vi "SubVI_Clamp #.vi"(8 "error in":errorcluster, 10 "Parameter_Edge":T3={"ROI Descriptor"={"Global Rectangle"=[], "Contours"=[]}, "Edge Options"={"Edge Options"={"Edge Polarity"=0, "Kernel Size"=3, "Width"=3, "Minimum Edge Strength"=10.0, "Interpolation Type"=enum."Bilinear Fixed", "Data Processing Method"=enum."Average"}, "Scan Direction"=0, "Step Size"=5, "SD"=0.0, "Auto"=FALSE}, "條件(Clamp)"={"間距"=5.0}} {"ROI Descriptor"."Contours"."Type" items=["No Selection", "Point", "Line", "Rectangle", "Oval", "Polygon", "Free", "Annulus", "Unused2", "Unused3", "Broken Line", "Free Hand Line", "Rotated Rectangle"]; "Edge Options"."Edge Options"."Edge Polarity" items=["All Edges", "Rising Edges", "Falling Edges"]; "Edge Options"."Edge Options"."Minimum Edge Strength" format="%.2f"; "Edge Options"."Edge Options"."Width" step=2; "Edge Options"."Edge Options"."Kernel Size" step=2; "Edge Options"."Scan Direction" items=["Left To Right", "Right To Left", "Top To Bottom", "Bottom To Top"]}, 11 "Image in":T2) -> (0 "error out":errorcluster, 1 "Distance":dbl, 2 "Perpendicular Line(Offset)":T1, 3 "Image Out":T2, 4 "Fit Line 2":T1, 6 "Fit Line":T1)   [LabVIEW 2013]
uses:
  <vilib>/vision/Image Controls.llb/IMAQ Image.ctl
  Control/Control_Clamp.ctl
  <vilib>/vision/Measure.llb/Edge Options.ctl
  <vilib>/vision/Measure.llb/Edge Polarity.ctl
  <vilib>/vision/NI_Vision_Development_Module.lvlib
  <vilib>/Analysis/NI_AALBase.lvlib
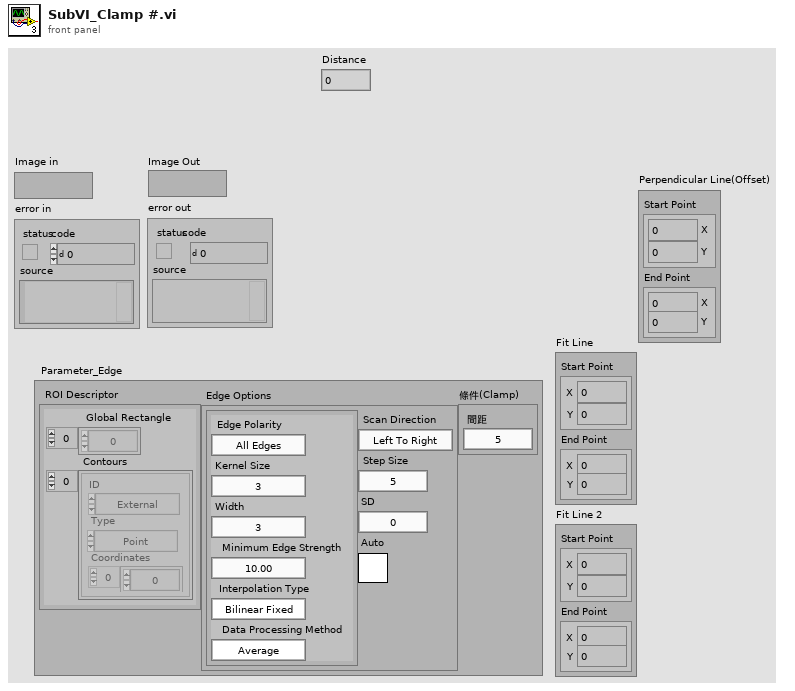
[diagram p1: front panel]
types:
  T1 = cluster{"Start Point":cluster{"X":sgl, "Y":sgl}, "End Point":cluster{"X":sgl, "Y":sgl}}
  T2 = typedef "IMAQ Image.ctl" = refnum<image>
  T3 = typedef "Control_Clamp.ctl" = cluster{"ROI Descriptor":cluster{"Global Rectangle":i32[], "Contours":cluster{"ID":enum32{"External", "Internal"}, "Type":u32, "Coordinates":i32[]}[]}, "Edge Options":cluster{"Edge Options":T4, "Scan Direction":u16, "Step Size":u32, "SD":dbl, "Auto":bool}, "條件(Clamp)":cluster{"間距":dbl}}
  T4 = typedef "Edge Options.ctl" = cluster{"Edge Polarity":T5, "Kernel Size":u32, "Width":u32, "Minimum Edge Strength":sgl, "Interpolation Type":enum32{"Zero Order", "Bilinear", "Quadratic", "Cubic", "Bilinear Fixed"}, "Data Processing Method":enum32{"Average", "Median"}}
  T5 = typedef "Edge Polarity.ctl" = u32
  T6 = cluster{"Global Rectangle":i32[], "Contours":cluster{"ID":enum32{"External", "Internal"}, "Type":u32, "Coordinates":i32[]}[]}
  T7 = cluster{"Edge Options":T4, "Scan Direction":u16, "Step Size":u32, "SD":dbl, "Auto":bool}
  T8 = cluster{"Point 1":cluster{"X":sgl, "Y":sgl}, "Point 2":cluster{"X":sgl, "Y":sgl}}
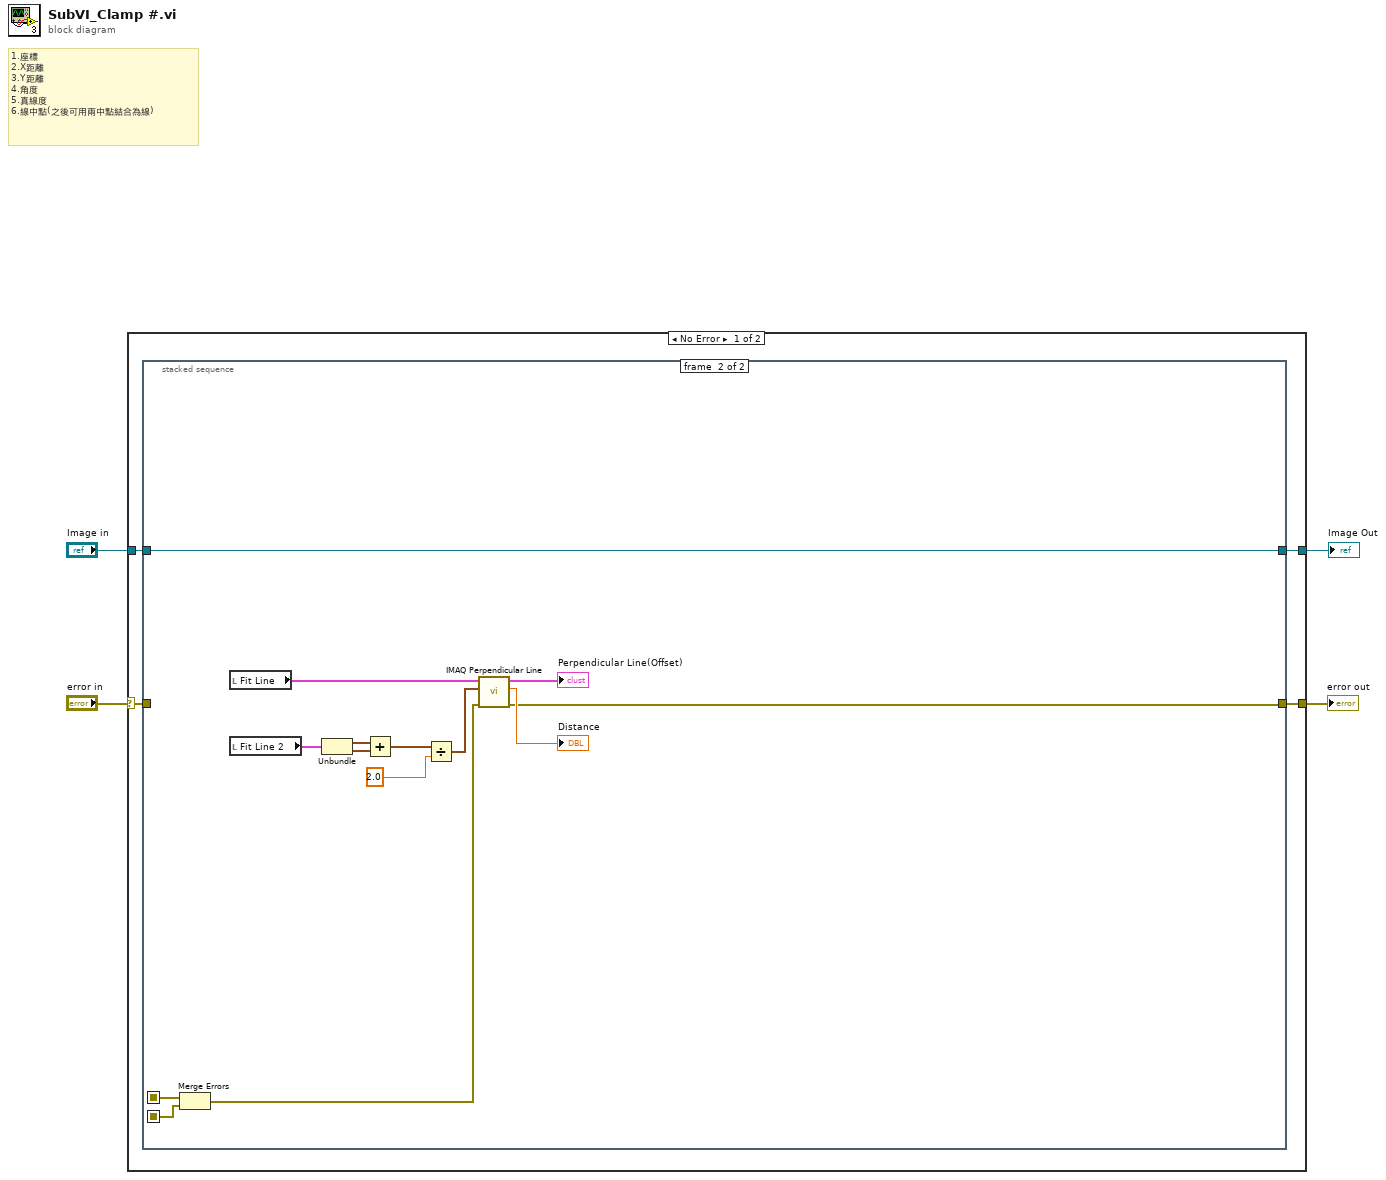
[diagram p0: block diagram]
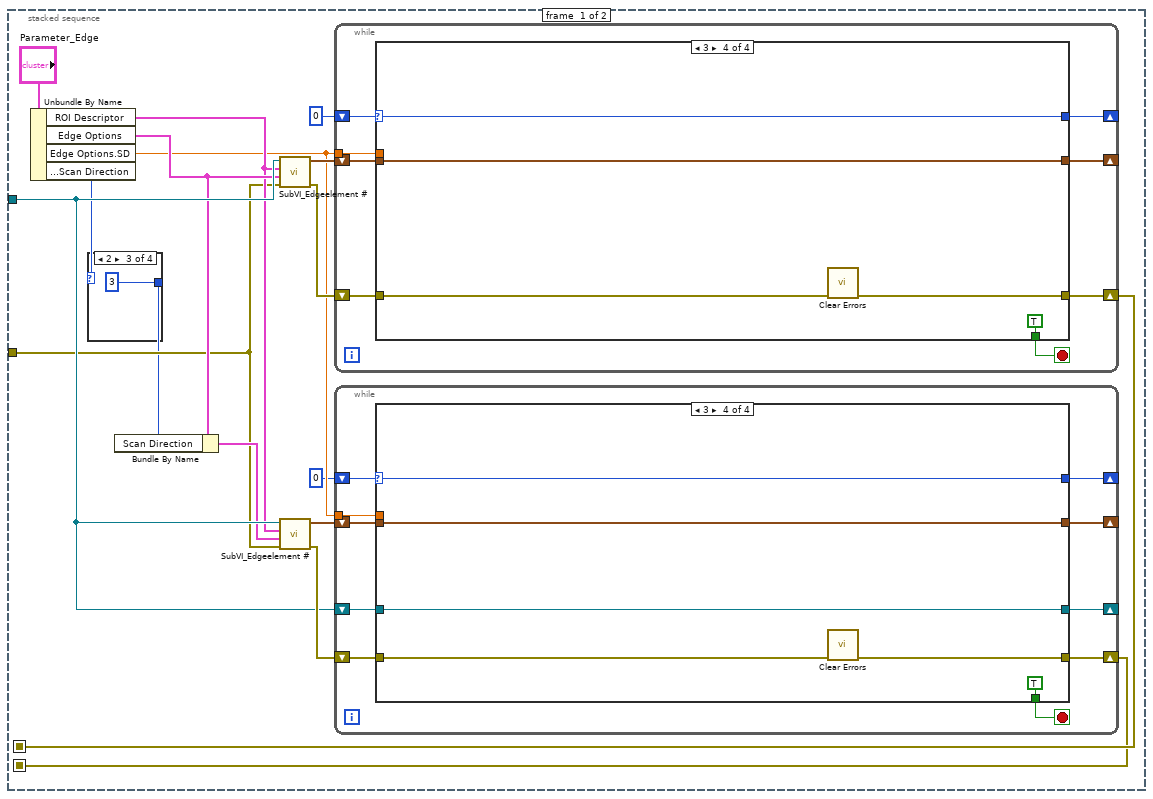
[diagram p2: hidden frame]
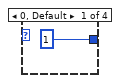
[diagram p3: hidden frame]
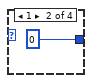
[diagram p4: hidden frame]
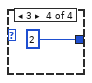
[diagram p5: hidden frame]
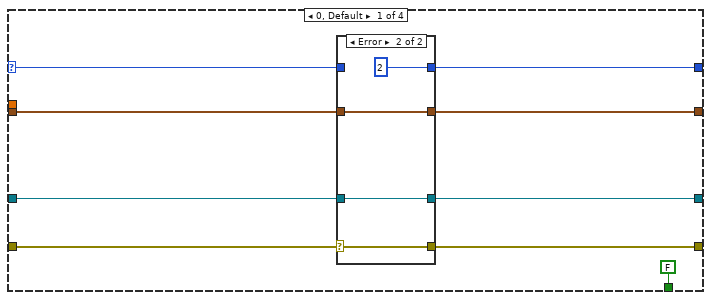
[diagram p6: hidden frame]
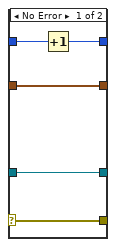
[diagram p7: hidden frame]
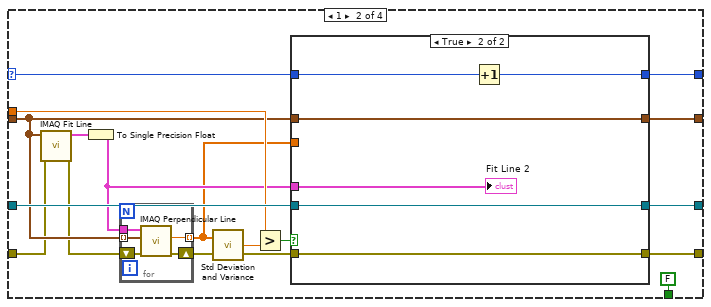
[diagram p8: hidden frame]
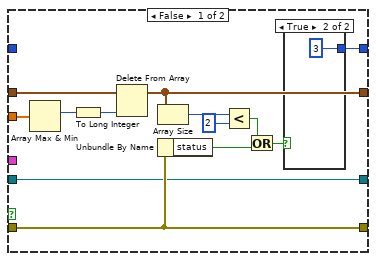
[diagram p9: hidden frame]
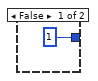
[diagram p10: hidden frame]
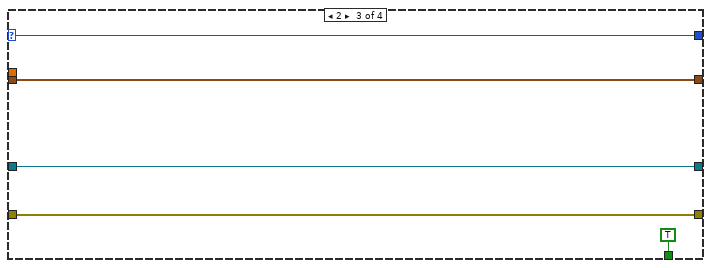
[diagram p11: hidden frame]
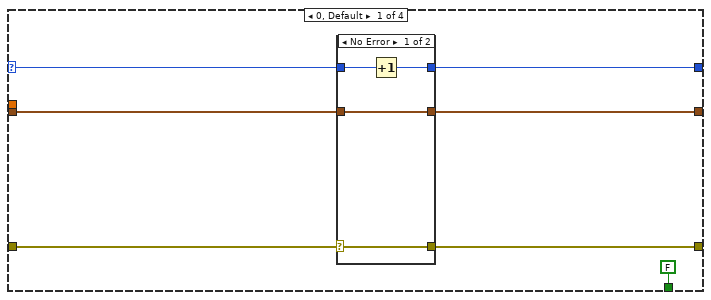
[diagram p12: hidden frame]
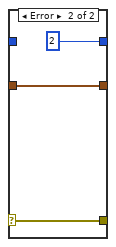
[diagram p13: hidden frame]
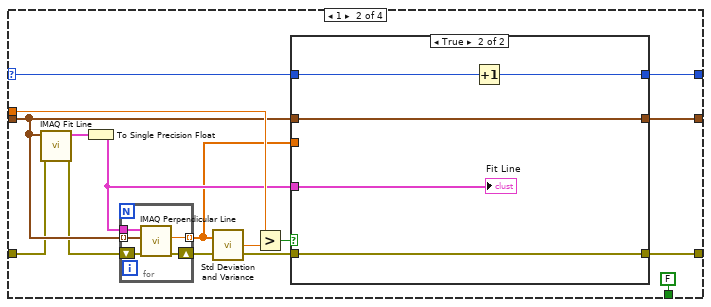
[diagram p14: hidden frame]
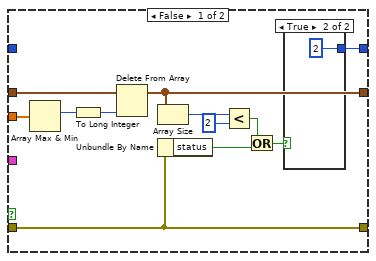
[diagram p15: hidden frame]
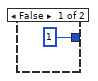
[diagram p16: hidden frame]
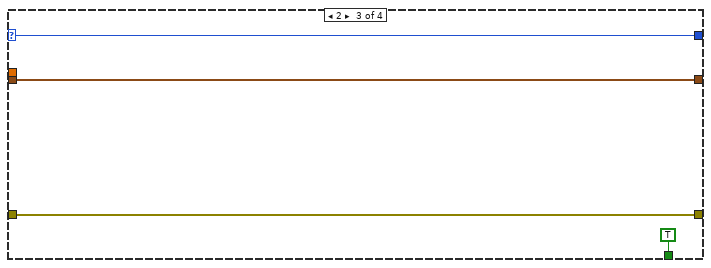
[diagram p17: hidden frame]
diagram:
  # "1.座標\n2.X距離\n3.Y距離\n4.角度\n5.真線度\n6.線中點(之後可用兩中點結合為線)"
  n1 = case shown="No Error" "error in" {
    selector: "error in" -> [w5 w197]
    tunnel: "Image in" -> [w6 w196]
    tunnel: [w8 w197] -> w2
    tunnel: [w7 w196] -> w1
    frame No Error {
      n2 = stacked-sequence {
        seq-local: [w10 _] -> [_ w184]
        seq-local: [w9 _] -> [_ w183]
        tunnel: [_ w185] -> w8
        tunnel: [_ w195] -> w7
        tunnel: w6 -> [w20 w195]
        tunnel: w5 -> [w16 _]
        frame #0 {
          n3 = Unbundle By Name("Parameter_Edge") -> ("ROI Descriptor"=w17:T6, "Edge Options"=w19:T7, "Edge Options.SD"=w13:dbl, "Edge Options.Scan Direction"=w15:u16)
          n4 = case shown="2" w15 {
            tunnel: [u16 1 u16 0 u16 3 u16 2] -> w14
            frame 0, Default {
            }
            frame 1 {
            }
            frame 2 {
            }
            frame 3 {
            }
          }
          n5 = Bundle By Name(cluster=w19, "Scan Direction"=w14) -> (w18:T7)
          n6 = call "SubVI_Edgeelement #.vi"("Error In"=w16, "Parameter_Edge"=w19, "ROI Descriptor"=w17, "Image In"=w20) -> ("Error Out"=w24:errorcluster, "Location"=w22:cluster{"X":sgl, "Y":sgl}[])  [unwired: 4 in, 2 out]
          n7 = call "SubVI_Edgeelement #.vi"("Error In"=w16, "Parameter_Edge"=w18, "ROI Descriptor"=w17, "Image In"=w20) -> ("Error Out"=w21:errorcluster, "Location"=w12:cluster{"X":sgl, "Y":sgl}[])  [unwired: 4 in, 2 out]
          n8 = while {
            shift-right: [w117] -> _
            shift-left: 0 -> [w119]
            shift-right: [w116] -> w10
            shift-left: w24 -> [w118]
            shift-right: [w114] -> _
            shift-left: w22 -> [w115]
            tunnel: w13 -> [w112]
            stop <- w113 stop-if-true
            n9 = case shown="3" w119 {
              selector: w119 -> [w124 w142 w174 w177]
              tunnel: w118 -> [w122 w135 w176 w181]
              tunnel: [w123 w143 w174 w177] -> w117
              tunnel: [w126 w144 w176 w180] -> w116
              tunnel: [w120 w146 w175 w179] -> w114
              tunnel: w115 -> [w121 w136 w175 w179]
              tunnel: [FALSE FALSE TRUE TRUE] -> w113
              tunnel: w112 -> [_ w140 _ _]
              frame 0, Default {
                n10 = case shown="No Error" w122 {
                  selector: w122 -> [w127 w132]
                  tunnel: [w127 w132] -> w126
                  tunnel: w124 -> [w130 _]
                  tunnel: [w129 2] -> w123
                  tunnel: w121 -> [w128 w131]
                  tunnel: [w128 w131] -> w120
                  frame No Error {
                    n11 = Increment(x=w130) -> (x+1=w129:i32)
                  }
                  frame Error {
                  }
                }
              }
              frame 1 {
                n12 = call "IMAQ Fit Line"("error in (no error)"=w135, "Points"=w136) -> ("error out"=w134:errorcluster, "Line Segment"=w139:T8)  [unwired: 4 in, 4 out]
                n13 = To Single Precision Float(number=w139) -> (single precision float=w138:T8)
                n14 = for {
                  tunnel: w138 -> [w172]
                  tunnel: w136 -> [w171] mode=indexing
                  tunnel: [w170] -> w137 mode=indexing
                  shift-right: [w168] -> w145
                  shift-left: w134 -> [w169]
                  n15 = call "IMAQ Perpendicular Line"("error in (no error)"=w169, "Point"=w171, "Line"=w172) -> ("error out"=w168:errorcluster, "Distance"=w170:dbl)  [unwired: 6 in, 1 out]
                }
                n16 = call <vilib>:"Std Deviation and Variance.vi"("X"=w137) -> ("standard deviation"=w148:dbl)  [unwired: 1 in, 2 out]
                n17 = Greater?(x=w140, y=w148) -> (0:w147:bool)
                n18 = case shown="True" w147 {
                  tunnel: w136 -> [w160 w165]
                  tunnel: [w156 w165] -> w146
                  tunnel: w145 -> [w151 w164]
                  tunnel: [w151 w164] -> w144
                  tunnel: [w158 w166] -> w143
                  tunnel: w142 -> [_ w167]
                  tunnel: w138 -> [_ w163]
                  tunnel: w137 -> [w149 _]
                  frame False {
                    n19 = Array Max & Min(array=w149) -> (max index (indices)=w159:i32)  [unwired: 3 out]
                    n20 = To Long Integer(number=w159) -> (32bit integer=w150:i32)
                    n21 = Delete From Array(array=w160, index=w150) -> (array with subset deleted=w156:cluster{"X":sgl, "Y":sgl}[])  [unwired: 1 in, 1 out]
                    n22 = Array Size(array=w156) -> (size(s)=w155:i32)
                    n23 = Unbundle By Name(w151) -> ("status"=w157:bool)
                    n24 = Less?(x=w155, y=2) -> (x < y?=w153:bool)
                    n25 = Or(x=w153, y=w157) -> (x .or. y?=w152:bool)
                    n26 = case shown="True" w152 {
                      tunnel: [1 2] -> w158
                      frame False {
                      }
                      frame True {
                      }
                    }
                  }
                  frame True {
                    n27 = Increment(x=w167) -> (x+1=w166:i32)
                    "Fit Line" <- w163
                  }
                }
              }
              frame 2 {
              }
              frame 3 {
                n28 = call <vilib>:"Clear Errors.vi"("error in (no error)"=w181) -> ("error out"=w180:errorcluster)  [unwired: 6 in]
              }
            }
          }
          n29 = while {
            shift-right: [w37] -> _
            shift-left: 0 -> [w39]
            shift-right: [w36] -> w9
            shift-left: w21 -> [w38]
            shift-right: [w34] -> _
            shift-left: w12 -> [w35]
            shift-right: [w32] -> _
            shift-left: w20 -> [w33]
            tunnel: w13 -> [w30]
            stop <- w31 stop-if-true
            n30 = case shown="3" w39 {
              selector: w39 -> [w44 w66 w102 w106]
              tunnel: w38 -> [w42 w59 w105 w111]
              tunnel: [w43 w67 w102 w106] -> w37
              tunnel: [w46 w68 w105 w110] -> w36
              tunnel: [w40 w72 w103 w108] -> w34
              tunnel: w35 -> [w41 w60 w103 w108]
              tunnel: w33 -> [w48 w71 w104 w109]
              tunnel: [w47 w70 w104 w109] -> w32
              tunnel: [FALSE FALSE TRUE TRUE] -> w31
              tunnel: w30 -> [_ w64 _ _]
              frame 0, Default {
                n31 = case shown="Error" w42 {
                  selector: w42 -> [w50 w55]
                  tunnel: w48 -> [w49 w56]
                  tunnel: [w49 w56] -> w47
                  tunnel: [w50 w55] -> w46
                  tunnel: w44 -> [w53 _]
                  tunnel: [w52 2] -> w43
                  tunnel: w41 -> [w51 w54]
                  tunnel: [w51 w54] -> w40
                  frame No Error {
                    n32 = Increment(x=w53) -> (x+1=w52:i32)
                  }
                  frame Error {
                  }
                }
              }
              frame 1 {
                n33 = call "IMAQ Fit Line"("error in (no error)"=w59, "Points"=w60) -> ("error out"=w58:errorcluster, "Line Segment"=w63:T8)  [unwired: 4 in, 4 out]
                n34 = To Single Precision Float(number=w63) -> (single precision float=w62:T8)
                n35 = for {
                  tunnel: w62 -> [w100]
                  tunnel: w60 -> [w99] mode=indexing
                  tunnel: [w98] -> w61 mode=indexing
                  shift-right: [w96] -> w69
                  shift-left: w58 -> [w97]
                  n36 = call "IMAQ Perpendicular Line"("error in (no error)"=w97, "Point"=w99, "Line"=w100) -> ("error out"=w96:errorcluster, "Distance"=w98:dbl)  [unwired: 6 in, 1 out]
                }
                n37 = call <vilib>:"Std Deviation and Variance.vi"("X"=w61) -> ("standard deviation"=w74:dbl)  [unwired: 1 in, 2 out]
                n38 = Greater?(x=w64, y=w74) -> (0:w73:bool)
                n39 = case shown="True" w73 {
                  tunnel: w60 -> [w87 w93]
                  tunnel: [w83 w93] -> w72
                  tunnel: w71 -> [w77 w92]
                  tunnel: [w77 w92] -> w70
                  tunnel: w69 -> [w78 w91]
                  tunnel: [w78 w91] -> w68
                  tunnel: [w85 w94] -> w67
                  tunnel: w66 -> [_ w95]
                  tunnel: w62 -> [_ w90]
                  tunnel: w61 -> [w75 _]
                  frame False {
                    n40 = Array Max & Min(array=w75) -> (max index (indices)=w86:i32)  [unwired: 3 out]
                    n41 = To Long Integer(number=w86) -> (32bit integer=w76:i32)
                    n42 = Delete From Array(array=w87, index=w76) -> (array with subset deleted=w83:cluster{"X":sgl, "Y":sgl}[])  [unwired: 1 in, 1 out]
                    n43 = Array Size(array=w83) -> (size(s)=w82:i32)
                    n44 = Unbundle By Name(w78) -> ("status"=w84:bool)
                    n45 = Less?(x=w82, y=2) -> (x < y?=w80:bool)
                    n46 = Or(x=w80, y=w84) -> (x .or. y?=w79:bool)
                    n47 = case shown="True" w79 {
                      tunnel: [1 3] -> w85
                      frame False {
                      }
                      frame True {
                      }
                    }
                  }
                  frame True {
                    n48 = Increment(x=w95) -> (x+1=w94:i32)
                    "Fit Line 2" <- w90
                  }
                }
              }
              frame 2 {
              }
              frame 3 {
                n49 = call <vilib>:"Clear Errors.vi"("error in (no error)"=w111) -> ("error out"=w110:errorcluster)  [unwired: 6 in]
              }
            }
          }
        }
        frame #1 {
          n50 = Merge Errors(w184, w183) -> (w182:errorcluster)
          n51 = local read "Fit Line"() -> (w188:T1)
          n52 = local read "Fit Line 2"() -> (w194:T1)
          n53 = Unbundle(w194) -> ("Start Point"=w193:cluster{"X":sgl, "Y":sgl}, "End Point"=w192:cluster{"X":sgl, "Y":sgl})
          n54 = Add(x=w193, y=w192) -> (x+y=w191:cluster{"X":sgl, "Y":sgl})
          n55 = Divide(x=w191, y=sgl 2.0) -> (x/y=w189:cluster{"X":sgl, "Y":sgl})
          n56 = call "IMAQ Perpendicular Line"("error in (no error)"=w182, "Point"=w189, "Line"=w188) -> ("error out"=w185:errorcluster, "Distance"=→"Distance":dbl, "Perpendicular Line"=→"Perpendicular Line(Offset)":T8)  [unwired: 6 in]
        }
      }
    }
    frame Error {
    }
  }
  "error out" <- w2
  "Image Out" <- w1
